vi "dfd_PR Cosine-Modulated Prototype Filter Design.vi"(7 "M":i32=4, 8 "error in (no error)":errorcluster, 10 "roll off":dbl=0.99, 11 "order":i32=39) -> (0 "error out":errorcluster, 3 "h":dbl[](array[numeric]))   [LabVIEW 2017, in "NI_DigFilter_FilterBank.lvlib"]
uses:
  <vilib>/addons/Digital Filter Design/NI_DigFilter_FilterBank.lvlib
  <vilib>/gmath/NumericalOptimization/stopping criteria.ctl
  <vilib>/gmath/NumericalOptimization/Quasi Newton.vi
  <vilib>/gmath/NI_Gmath.lvlib
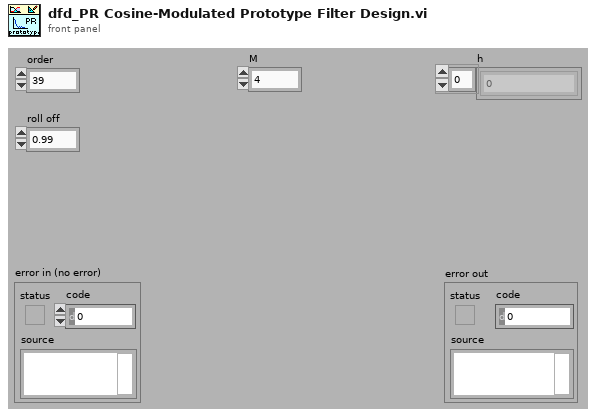
[diagram p1: front panel]
types:
  T1 = typedef "NI_Gmath.lvlib/stopping criteria.ctl" = cluster{"function tolerance":dbl, "parameter tolerance":dbl, "max iterations":i32, "max function calls":i32, "gradient tolerance":dbl, "max time (sec)":dbl}
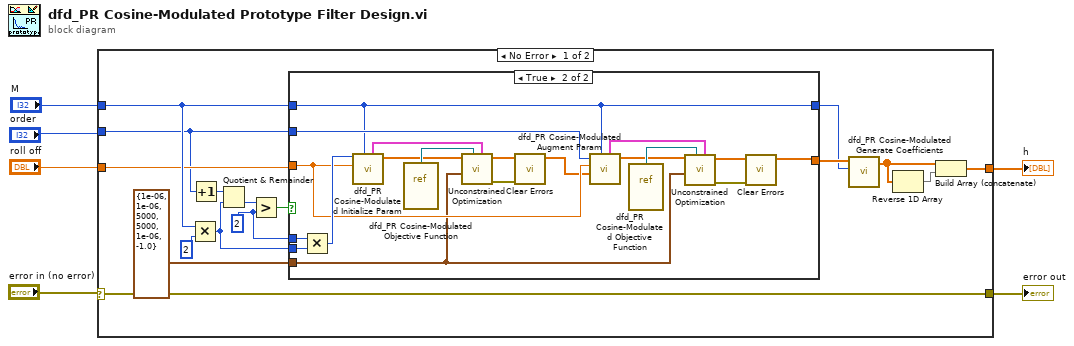
[diagram p0: block diagram]
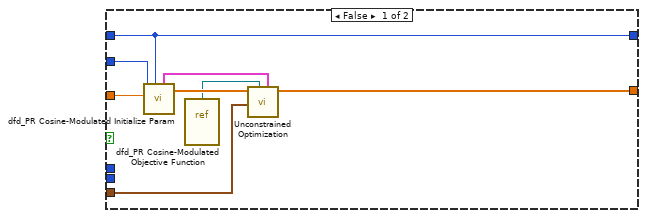
[diagram p2: hidden frame]
diagram:
  n1 = case shown="No Error" "error in (no error)" {
    selector: "error in (no error)" -> [w9 w48]
    tunnel: [w9 w48] -> w5
    tunnel: "M" -> [w18 _]
    tunnel: "order" -> [w7 _]
    tunnel: "roll off" -> [w8 _]
    tunnel: [w14 _] -> w1
    frame No Error {
      w13 = 2
      n2 = Multiply(x=w18, y=2) -> (x*y=w12:i32)
      n3 = Increment(x=w7) -> (x+1=w22:i32)
      n4 = Quotient & Remainder(x=w22, y=w12) -> (floor(x/y)=w20:i32)  [unwired: 1 out]
      n5 = Greater?(x=w20, y=w13) -> (0:w19:bool)
      n6 = case shown="True" w19 {
        tunnel: w18 -> [w24 w39]
        tunnel: w7 -> [w30 w42]
        tunnel: w8 -> [w29 w41]
        tunnel: [w25 w31] -> w17
        tunnel: [w24 w39] -> w16
        tunnel: w13 -> [_ w47]
        tunnel: w12 -> [_ w46]
        tunnel: T1 {"function tolerance"=1e-06, "parameter tolerance"=1e-06, "max iterations"=5000, "max function calls"=5000, "gradient tolerance"=1e-06, "max time (sec)"=-1.0} ("stopping criteria") -> [w23 w33]
        frame False {
          n7 = call <vilib>:"dfd_PR Cosine-Modulated Initialize Param.vi"("M"=w24, "roll off"=w29, "order"=w30) -> ("Initial phi"=w28:dbl[], "param"=w27:cluster{"M":i32, "Us":dbl[][], "roll off":dbl})  [unwired: 7 in]
          n8 = vi-ref <vilib>:"dfd_PR Cosine-Modulated Objective Function.vi"() -> (w26:refnum<vi>)
          n9 = call-poly <vilib>:"Unconstrained Optimization.vi"("function data"=w27, "objective function"=w26, "stopping criteria"=w23, "start"=w28) -> ("minimum"=w25:dbl[])  [unwired: 4 in, 3 out]
        }
        frame True {
          n10 = Multiply(x=w47, y=w46) -> (x*y=w45:i32)
          n11 = call <vilib>:"dfd_PR Cosine-Modulated Initialize Param.vi"("M"=w39, "roll off"=w41, "order"=w45) -> ("Initial phi"=w43:dbl[], "param"=w35:cluster{"M":i32, "Us":dbl[][], "roll off":dbl})  [unwired: 7 in]
          n12 = vi-ref <vilib>:"dfd_PR Cosine-Modulated Objective Function.vi"() -> (w44:refnum<vi>)
          n13 = call-poly <vilib>:"Unconstrained Optimization.vi"("function data"=w35, "objective function"=w44, "stopping criteria"=w33, "start"=w43) -> ("error out"=w36:errorcluster, "minimum"=w32:dbl[])  [unwired: 4 in, 2 out]
          n14 = call <vilib>:"Clear Errors.vi"("error in (no error)"=w36) -> ()  [unwired: 5 in, 2 out]
          n15 = call <vilib>:"dfd_PR Cosine-Modulated Augment Param.vi"("M"=w39, "Initial phi"=w32, "roll off"=w41, "order"=w42) -> ("Augmented phi"=w38:dbl[], "param"=w34:cluster{"M":i32, "Us":dbl[][], "roll off":dbl})  [unwired: 6 in]
          n16 = vi-ref <vilib>:"dfd_PR Cosine-Modulated Objective Function.vi"() -> (w40:refnum<vi>)
          n17 = call-poly <vilib>:"Unconstrained Optimization.vi"("function data"=w34, "objective function"=w40, "stopping criteria"=w33, "start"=w38) -> ("error out"=w37:errorcluster, "minimum"=w31:dbl[])  [unwired: 4 in, 2 out]
          n18 = call <vilib>:"Clear Errors.vi"("error in (no error)"=w37) -> ()  [unwired: 5 in, 2 out]
        }
      }
      n19 = call <vilib>:"dfd_PR Cosine-Modulated Generate Coefficients.vi"("M"=w16, "phi"=w17) -> ("p"=w11:dbl[])  [unwired: 9 in]
      n20 = Reverse 1D Array(array=w11) -> (reversed array=w15:dbl[])
      n21 = Build Array (concatenate)(w11, w15) -> (w14:dbl[])
    }
    frame Error {
    }
  }
  "error out" <- w5
  "h" <- w1
